vi "test Write and Read Boolean Array.vi"(8 "error in (no error)":errorcluster, 11 "TestCase in":refnum<class "Read Value Tests.lvclass">) -> (0 "error out":errorcluster, 3 "TestCase out":refnum<class "Read Value Tests.lvclass">)   [LabVIEW 2017, in "Pointer Tests.lvlib" / "Read Value Tests.lvclass"]
uses:
  Read Value Tests.lvclass
  Read Value Tests.lvclass/Read Value Tests.ctl
  Source/Classes/Pointer/Pointer.lvclass/Pointer.ctl
  Source/Classes/Pointer/Public/Read/Read (1D Bool).vi
  Source/Classes/Pointer/Public/Read (No Check)/Read (No Check 1D Bool).vi
  Source/Classes/Pointer/Protected/Parameter Checking/Check Null Pointer.vi
  Source/Classes/Pointer/Protected/Parameter Checking/Check Subset (Power of 2).vi
  Source/Classes/Pointer/API/Accessors/Get Address.vi
  Source/Classes/Pointer/Protected/Errors.vi
  Source/Classes/Pointer/Protected/Error VIs/Null Pointer.vi
  Source/Classes/Pointer/Protected/Error VIs/Out of Bounds.vi
  Source/Classes/Pointer/API/Accessors/Get Size.vi
  Source/Classes/Pointer/Private/Count to Size.vi
  Source/Classes/Pointer/Protected/Error Building/Create Error.vi
  Source/VIs/Write String into Source.vi
  Source/Classes/Pointer/Protected/Error Building/Write Pointer Size.vi
  Source/VIs/Write Number into Source.vi
  Source/VIs/VIs for Poly/Write U64 into Source.vi
  Source/Constants/Constants.vi
  Source/Constants/Library Name.vi
  Source/Classes/Pointer/Protected/Error Building/Get Error Info.vi
  Source/VIs/Create Error Cluster.vi
  Source/VIs/VIs for Poly/Create Error Cluster (256B).vi
  Source/VIs/Set Error Status.vi
  Source/VIs/Set Error Code.vi
  Source/VIs/Set Error Source.vi
  <vilib>/addons/_JKI Toolkits/VI Tester/TestCase.llb/TestCase.lvclass
  Source/Classes/Pointer/Pointer.lvclass
  C:/Program Files (x86)/National Instruments/LabVIEW 2017/vi.lib/addons/_JKI Toolkits/VI Tester/TestCase.llb/TestCase.lvclass
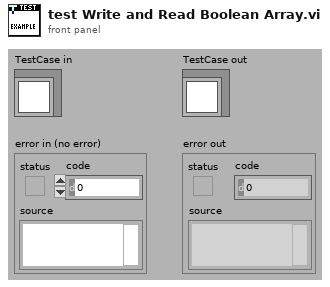
[diagram p1: front panel]
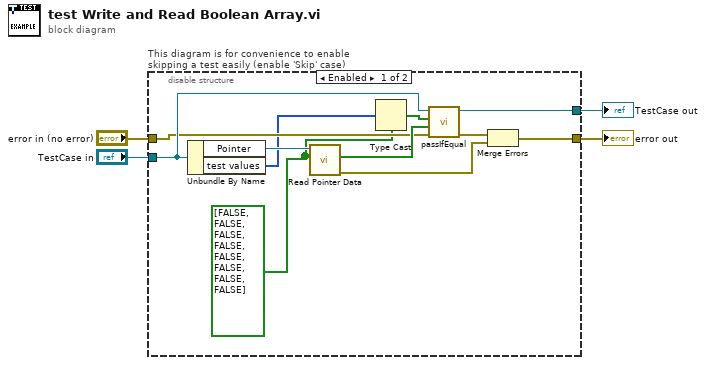
[diagram p0: block diagram]
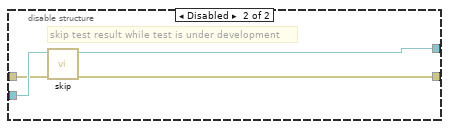
[diagram p2: hidden frame]
diagram:
  n1 = disable-structure "This diagram is for convenience to enable skipping a test easily (enable 'Skip' case)" shown="Enabled" {
    disable-tunnel: "TestCase in" -> [w13 w19]
    disable-tunnel: [w12 w17] -> w1
    disable-tunnel: [w9 w18] -> w3
    disable-tunnel: "error in (no error)" -> [w10 w16]
    frame Enabled {
      w5 = bool[] [FALSE, FALSE, FALSE, FALSE, FALSE, FALSE, FALSE, FALSE] ("buffer in")
      n2 = Unbundle By Name(w13) -> ("Pointer"=w14:refnum<class "Pointer.lvclass">, "test values"=w7:u8[])
      n3 = call-poly "Read Pointer Data.vi"("buffer in"=w5, "Pointer in"=w14) -> ("error out"=w8:errorcluster, "buffer out"=w15:bool[])  [unwired: 6 in, 2 out]
      n4 = Type Cast(type=w5, x=w7) -> (*(type *) &x=w6:bool[])
      n5 = call-dynamic "passIfEqual.vi"("error in (no error)"=w10, "y"=w15, "x"=w6, "TestCase in"=w13) -> ("error out"=w11:errorcluster, "TestCase out"=w12:refnum<class "Read Value Tests.lvclass">)  [unwired: 6 in]
      n6 = Merge Errors(w11, w8) -> (w9:errorcluster)
    }
    frame Disabled {
      # "skip test result while test is under development"
      n7 = call <vilib>:"skip.vi"("error in (no error)"=w16, "TestCase in"=w19) -> ("error out"=w18:errorcluster, "TestCase out"=w17:refnum<class "Read Value Tests.lvclass">)  [unwired: 8 in]
    }
  }
  "error out" <- w3
  "TestCase out" <- w1
